vi "Handle transmission status bytes.vi"(8 "error in":errorcluster, 10 "Data in":u8[](array[numeric]), 11 "All ROBs info cluster":T1) -> (0 "error out":errorcluster)   [LabVIEW 2016]
uses:
  Typedefs/All ROBs info cluster refnum.ctl
  Global Variables/Master Ready For Data.vi
  Global Variables/AllowUserMessages.vi
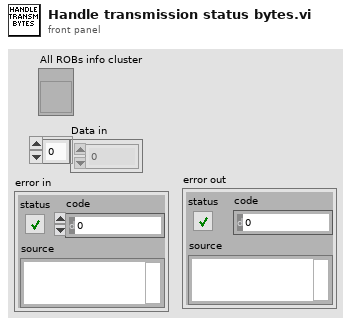
[diagram p1: front panel]
types:
  T1 = typedef "All ROBs info cluster refnum.ctl" = refnum<vi>
  T2 = typedef "ROB display info.ctl" = cluster{"ID:":i32, "State:":string, "Voltages":i32, "Temp:":dbl, "Latch count:":i32, "VRef:":enum16{"External", "Internal", "Unknown"}, "Trigthres:":i32, "MPPC EN":bool, "Test charge":bool, "Responding":bool, "Last update":timestamp}
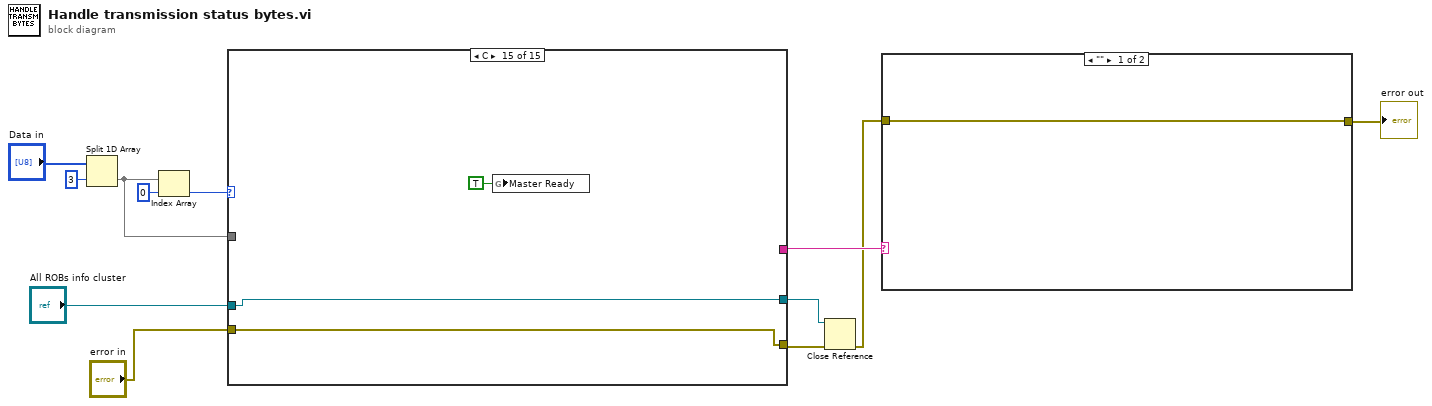
[diagram p0: block diagram]
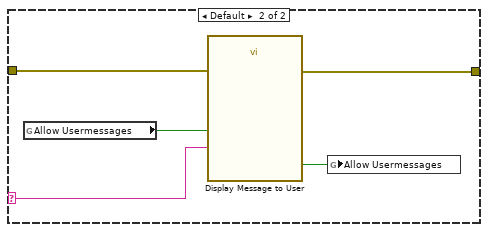
[diagram p2: hidden frame]
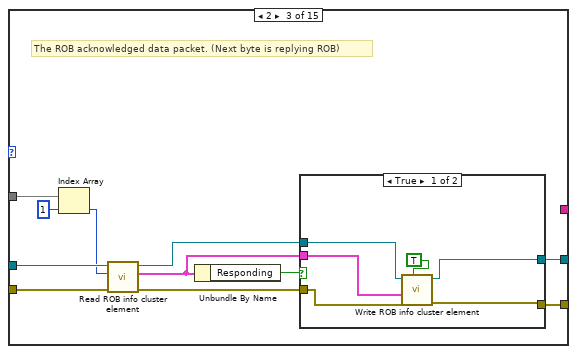
[diagram p5: hidden frame]
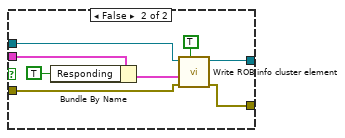
[diagram p6: hidden frame]
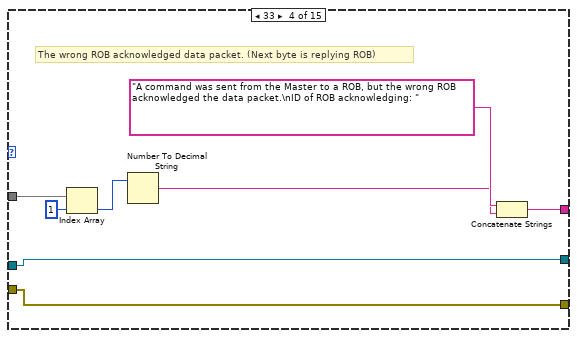
[diagram p7: hidden frame]
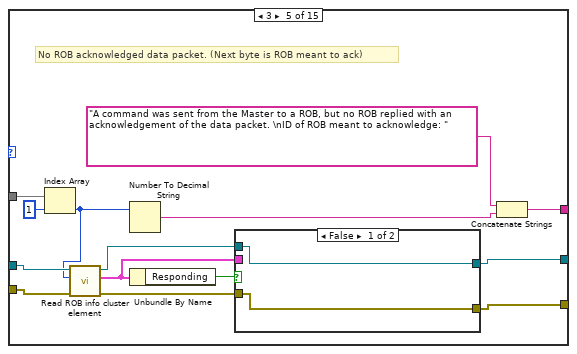
[diagram p8: hidden frame]
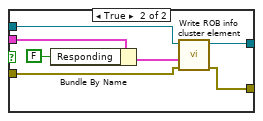
[diagram p9: hidden frame]
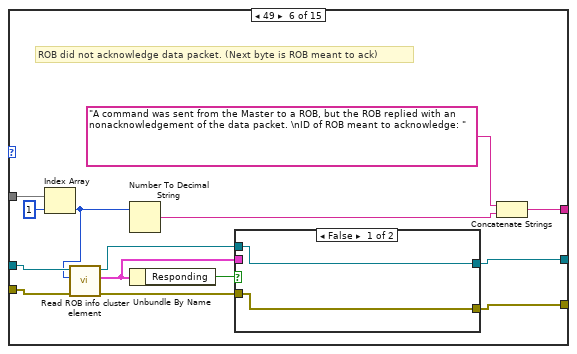
[diagram p10: hidden frame]
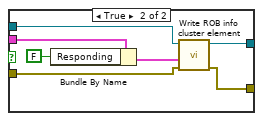
[diagram p11: hidden frame]
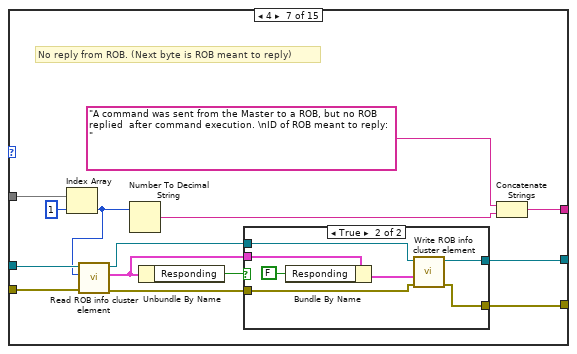
[diagram p12: hidden frame]
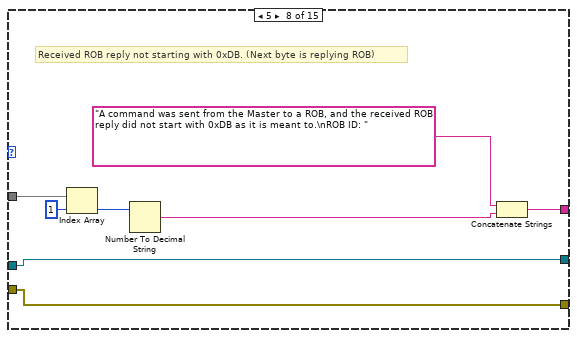
[diagram p14: hidden frame]
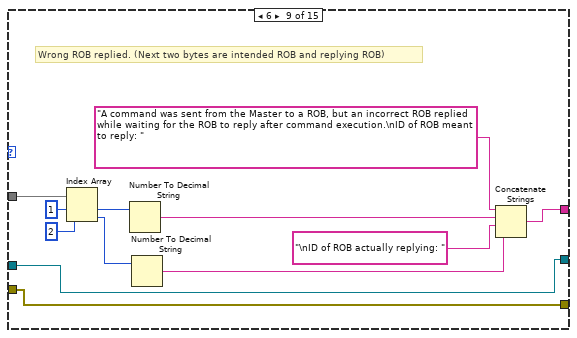
[diagram p15: hidden frame]
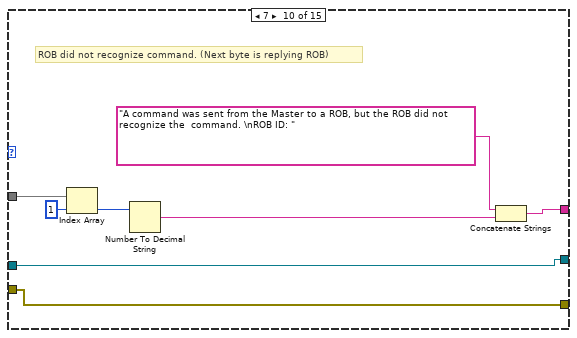
[diagram p16: hidden frame]
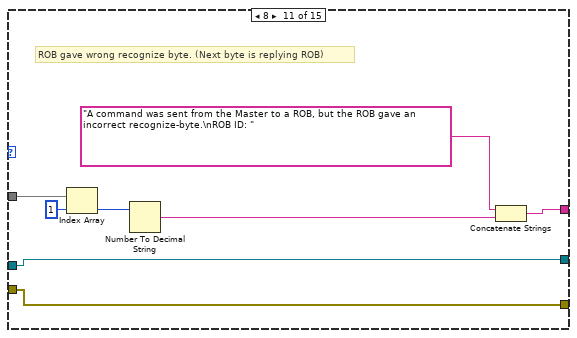
[diagram p17: hidden frame]
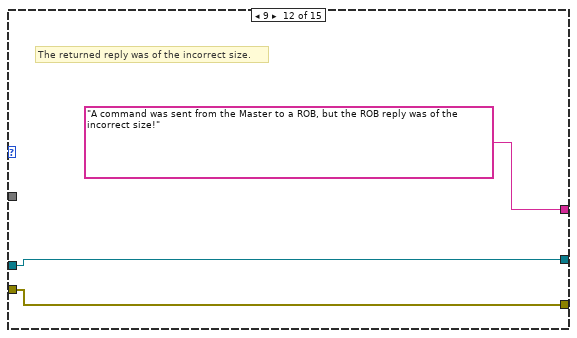
[diagram p18: hidden frame]
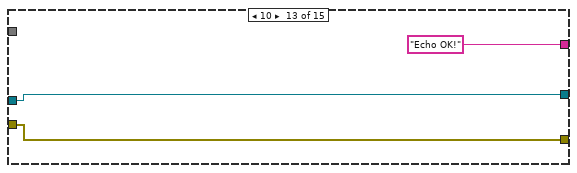
[diagram p19: hidden frame]
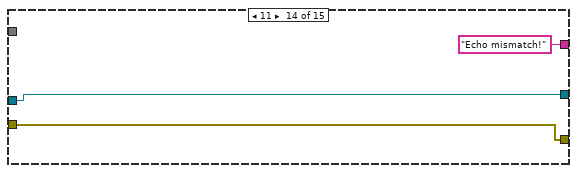
[diagram p20: hidden frame]
diagram:
  n1 = Split 1D Array(array="Data in", index=3) -> (second subarray=w8:u8[])  [unwired: 1 out]
  n2 = Index Array(array=w8, index=0) -> (element=w9:u8)
  n3 = case shown="C" w9 {
    tunnel: w8 -> [_ _ w18 w48 w62 w85 w108 w125 w137 w145 w153 _ _ _ _]
    tunnel: [_ _ _ w44 w59 w82 w105 w121 w133 w141 w149 "A command was sent from the Master to a ROB, but the ROB reply was of the incorrect size!" "Echo OK!" "Echo mismatch!" _] -> w3
    tunnel: "All ROBs info cluster" -> [w14 w15 w27 w42 w53 w76 w99 w119 w127 w140 w148 w156 w159 w162 w166]
    tunnel: "error in" -> [w13 w16 w26 w43 w54 w77 w100 w120 w128 w139 w147 w155 w158 w161 w165]
    tunnel: [w13 w16 w21 w43 w52 w75 w98 w120 w128 w139 w147 w155 w158 w161 w165] -> w5
    tunnel: [w14 w15 w20 w42 w51 w74 w97 w119 w127 w140 w148 w156 w159 w162 w166] -> w4
    frame 0, Default {
      # "This case is already taken care of by SendSerialData\nin the main VI state machine."
      # "Master recognized data packet"
    }
    frame 1 {
      # "This case is already taken care of by SendSerialData\nin the main VI state machine."
      # "Master did not recognize data packet"
    }
    frame 2 {
      # "The ROB acknowledged data packet. (Next byte is replying ROB)"
      n4 = Index Array(array=w18, index=1) -> (element=w17:u8)
      n5 = call "Read ROB info cluster element.vi"("error in (no error)"=w26, "Channel"=w17, "ROB info clusters"=w27) -> ("error out"=w22:errorcluster, "ROB Info-display"=w24:T2, "ROB info clusters"=w23:T1)  [unwired: 5 in, 1 out]
      n6 = Unbundle By Name(w24) -> ("Responding"=w25:bool)
      n7 = case shown="True" w25 {
        tunnel: w24 -> [w28 w41]
        tunnel: w23 -> [w30 w38]
        tunnel: w22 -> [w32 w37]
        tunnel: [w31 w36] -> w21
        tunnel: [w29 w35] -> w20
        frame True {
          n8 = call "Write ROB info cluster element.vi"("Update timestamp (F)"=TRUE, "error in (no error)"=w32, "ROB Info-display"=w28, "Hist cluster"=w30) -> ("error out"=w31:errorcluster, "Hist cluster"=w29:T1)  [unwired: 6 in]
        }
        frame False {
          n9 = Bundle By Name(cluster=w41, "Responding"=TRUE) -> (w39:T2)
          n10 = call "Write ROB info cluster element.vi"("Update timestamp (F)"=TRUE, "error in (no error)"=w37, "ROB Info-display"=w39, "Hist cluster"=w38) -> ("error out"=w36:errorcluster, "Hist cluster"=w35:T1)  [unwired: 6 in]
        }
      }
    }
    frame 33 {
      # "The wrong ROB acknowledged data packet. (Next byte is replying ROB)"
      n11 = Index Array(array=w48, index=1) -> (element=w47:u8)
      n12 = Number To Decimal String(number=w47) -> (decimal integer string=w45:string)  [unwired: 1 in]
      n13 = Concatenate Strings("A command was sent from the Master to a ROB, but the wrong ROB acknowledged the data packet.\nID of ROB acknowledging: ", w45) -> (w44:string)
    }
    frame 3 {
      # "No ROB acknowledged data packet. (Next byte is ROB meant to ack)"
      n14 = Index Array(array=w62, index=1) -> (element=w50:u8)
      n15 = call "Read ROB info cluster element.vi"("error in (no error)"=w54, "Channel"=w50, "ROB info clusters"=w53) -> ("error out"=w55:errorcluster, "ROB Info-display"=w57:T2, "ROB info clusters"=w56:T1)  [unwired: 5 in, 1 out]
      n16 = Number To Decimal String(number=w50) -> (decimal integer string=w60:string)  [unwired: 1 in]
      n17 = Unbundle By Name(w57) -> ("Responding"=w58:bool)
      n18 = case shown="False" w58 {
        tunnel: w57 -> [_ w72]
        tunnel: w56 -> [w65 w69]
        tunnel: w55 -> [w64 w68]
        tunnel: [w64 w67] -> w52
        tunnel: [w65 w66] -> w51
        frame False {
        }
        frame True {
          n19 = Bundle By Name(cluster=w72, "Responding"=FALSE) -> (w70:T2)
          n20 = call "Write ROB info cluster element.vi"("error in (no error)"=w68, "ROB Info-display"=w70, "Hist cluster"=w69) -> ("error out"=w67:errorcluster, "Hist cluster"=w66:T1)  [unwired: 7 in]
        }
      }
      n21 = Concatenate Strings("A command was sent from the Master to a ROB, but no ROB replied with an acknowledgement of the data packet. \nID of ROB meant to acknowledge: ", w60) -> (w59:string)
    }
    frame 49 {
      # "ROB did not acknowledge data packet. (Next byte is ROB meant to ack)"
      n22 = Index Array(array=w85, index=1) -> (element=w73:u8)
      n23 = call "Read ROB info cluster element.vi"("error in (no error)"=w77, "Channel"=w73, "ROB info clusters"=w76) -> ("error out"=w78:errorcluster, "ROB Info-display"=w80:T2, "ROB info clusters"=w79:T1)  [unwired: 5 in, 1 out]
      n24 = Number To Decimal String(number=w73) -> (decimal integer string=w83:string)  [unwired: 1 in]
      n25 = Unbundle By Name(w80) -> ("Responding"=w81:bool)
      n26 = case shown="False" w81 {
        tunnel: w80 -> [_ w95]
        tunnel: w79 -> [w88 w92]
        tunnel: w78 -> [w87 w91]
        tunnel: [w87 w90] -> w75
        tunnel: [w88 w89] -> w74
        frame False {
        }
        frame True {
          n27 = Bundle By Name(cluster=w95, "Responding"=FALSE) -> (w93:T2)
          n28 = call "Write ROB info cluster element.vi"("error in (no error)"=w91, "ROB Info-display"=w93, "Hist cluster"=w92) -> ("error out"=w90:errorcluster, "Hist cluster"=w89:T1)  [unwired: 7 in]
        }
      }
      n29 = Concatenate Strings("A command was sent from the Master to a ROB, but the ROB replied with an nonacknowledgement of the data packet. \nID of ROB meant to acknowledge: ", w83) -> (w82:string)
    }
    frame 4 {
      # "No reply from ROB. (Next byte is ROB meant to reply)"
      n30 = Index Array(array=w108, index=1) -> (element=w96:u8)
      n31 = call "Read ROB info cluster element.vi"("error in (no error)"=w100, "Channel"=w96, "ROB info clusters"=w99) -> ("error out"=w104:errorcluster, "ROB Info-display"=w102:T2, "ROB info clusters"=w103:T1)  [unwired: 5 in, 1 out]
      n32 = Number To Decimal String(number=w96) -> (decimal integer string=w106:string)  [unwired: 1 in]
      n33 = Unbundle By Name(w102) -> ("Responding"=w101:bool)
      n34 = case shown="True" w101 {
        tunnel: w102 -> [_ w118]
        tunnel: w103 -> [w111 w115]
        tunnel: w104 -> [w110 w114]
        tunnel: [w110 w113] -> w98
        tunnel: [w111 w112] -> w97
        frame False {
        }
        frame True {
          n35 = Bundle By Name(cluster=w118, "Responding"=FALSE) -> (w116:T2)
          n36 = call "Write ROB info cluster element.vi"("error in (no error)"=w114, "ROB Info-display"=w116, "Hist cluster"=w115) -> ("error out"=w113:errorcluster, "Hist cluster"=w112:T1)  [unwired: 7 in]
        }
      }
      n37 = Concatenate Strings("A command was sent from the Master to a ROB, but no ROB replied  after command execution. \nID of ROB meant to reply: ", w106) -> (w105:string)
    }
    frame 5 {
      # "Received ROB reply not starting with 0xDB. (Next byte is replying ROB)"
      n38 = Index Array(array=w125, index=1) -> (element=w124:u8)
      n39 = Number To Decimal String(number=w124) -> (decimal integer string=w122:string)  [unwired: 1 in]
      n40 = Concatenate Strings("A command was sent from the Master to a ROB, and the received ROB reply did not start with 0xDB as it is meant to.\nROB ID: ", w122) -> (w121:string)
    }
    frame 6 {
      # "Wrong ROB replied. (Next two bytes are intended ROB and replying ROB)"
      n41 = Index Array(array=w137, index #1=1 ("index"), index #2=2 ("index")) -> (element #1=w136:u8, element #2=w130:u8)
      n42 = Number To Decimal String(number=w136) -> (decimal integer string=w134:string)  [unwired: 1 in]
      n43 = Number To Decimal String(number=w130) -> (decimal integer string=w129:string)  [unwired: 1 in]
      n44 = Concatenate Strings("A command was sent from the Master to a ROB, but an incorrect ROB replied while waiting for the ROB to reply after command execution.\nID of ROB meant to reply: ", w134, "\nID of ROB actually replying: ", w129) -> (w133:string)
    }
    frame 7 {
      # "ROB did not recognize command. (Next byte is replying ROB)"
      n45 = Index Array(array=w145, index=1) -> (element=w144:u8)
      n46 = Number To Decimal String(number=w144) -> (decimal integer string=w142:string)  [unwired: 1 in]
      n47 = Concatenate Strings("A command was sent from the Master to a ROB, but the ROB did not recognize the  command. \nROB ID: ", w142) -> (w141:string)
    }
    frame 8 {
      # "ROB gave wrong recognize byte. (Next byte is replying ROB)"
      n48 = Index Array(array=w153, index=1) -> (element=w152:u8)
      n49 = Number To Decimal String(number=w152) -> (decimal integer string=w150:string)  [unwired: 1 in]
      n50 = Concatenate Strings("A command was sent from the Master to a ROB, but the ROB gave an incorrect recognize-byte.\nROB ID: ", w150) -> (w149:string)
    }
    frame 9 {
      # "The returned reply was of the incorrect size."
    }
    frame 10 {
    }
    frame 11 {
    }
    frame 12 {
      n51 = global write "Master Ready For Data.vi" "Master Ready"(TRUE ("Master Ready")) -> ()
    }
  }
  n52 = Close Reference(reference=w4, error in (no error)=w5) -> (error out=w2:errorcluster)
  n53 = case shown="\"\"" w3 {
    selector: w3 -> [_ w172]
    tunnel: w2 -> [w167 w169]
    tunnel: [w167 w168] -> w1
    frame "" {
    }
    frame Default {
      n54 = global read "AllowUserMessages.vi" "Allow Usermessages"() -> (w171:bool)
      n55 = call "Display Message to User"("error in (no error)"=w169, "Enable"=w171, "Message"=w172) -> ("error out"=w168:errorcluster, "OK"=w170:bool)  [unwired: 7 in]
      n56 = global write "AllowUserMessages.vi" "Allow Usermessages"(w170) -> ()
    }
  }
  "error out" <- w1
